vi "Set IP Address.vi"(8 "error in (no error)":errorcluster, 10 "IP Address":string, 11 "ENET in":refnum<class "ENET_BS120x.lvclass">) -> (0 "error out":errorcluster, 3 "ENET out":refnum<class "ENET_BS120x.lvclass">)   [LabVIEW 2021]
uses:
  ENET_BS120x.lvclass
  <vilib>/regexp/Match Regular Expression.xnode
  C:/Users/Public/Documents/Projects/7100-00109 SW BS1201 LV Driver/trunk/source/BS120x.lvclass
  C:/Users/Public/Documents/Projects/7100-00109 SW BS1201 LV Driver/trunk/source/ENET_BS120x/ENET_BS120x.lvclass
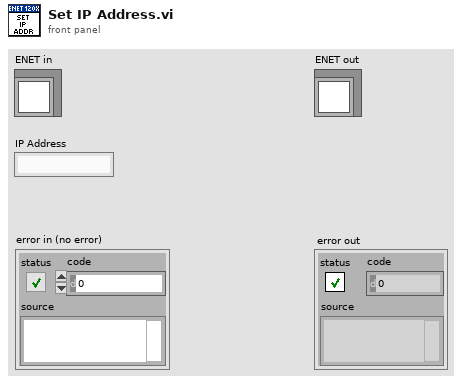
[diagram p1: front panel]
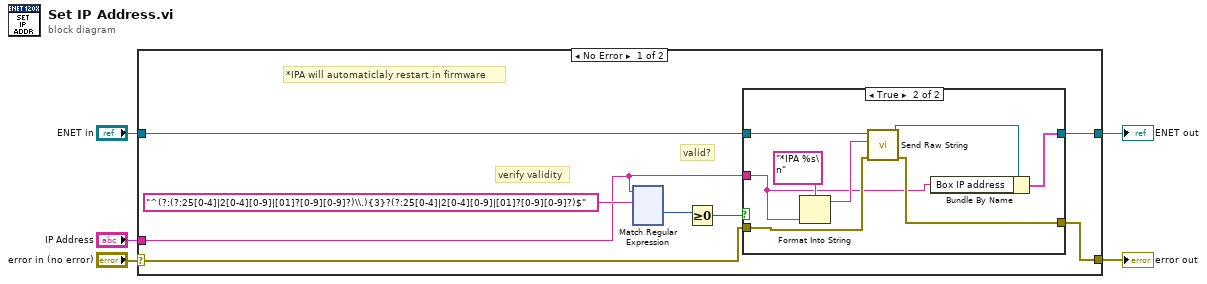
[diagram p0: block diagram]
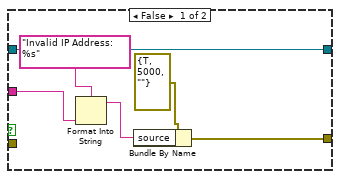
[diagram p2: hidden frame]
diagram:
  n1 = case shown="No Error" "error in (no error)" {
    selector: "error in (no error)" -> [w7 w146]
    tunnel: [w6 w146] -> w5
    tunnel: [w8 w145] -> w4
    tunnel: "ENET in" -> [w13 w145]
    tunnel: "IP Address" -> [w9 _]
    frame No Error {
      # "*IPA will automaticlaly restart in firmware"
      # "valid?"
      # "verify validity"
      n2 = xnode "Match Regular Expression"("input string"=w9, "regular expression"="^(?:(?:25[0-4]|2[0-4][0-9]|[01]?[0-9][0-9]?)\\.){3}?(?:25[0-4]|2[0-4][0-9]|[01]?[0-9][0-9]?)$") -> ("offset past match"=w11:i32)  [unwired: 4 in, 4 out]
      n3 = Greater Or Equal To 0?(x=w11) -> (x >= 0?=w10:bool)
      n4 = case shown="True" w10 {
        tunnel: w13 -> [w19 w27]
        tunnel: w9 -> [w17 w20]
        tunnel: [w19 w21] -> w8
        tunnel: w7 -> [_ w24]
        tunnel: [w14 w23] -> w6
        frame False {
          n5 = Format Into String(format string="Invalid IP Address: %s", w17) -> (resulting string=w15:string)  [unwired: 2 in, 1 out]
          n6 = Bundle By Name(cluster=errorcluster {"status"=TRUE, "code"=5000, "source"=""} ("error out"), "source"=w15) -> (w14:errorcluster)
        }
        frame True {
          n7 = Format Into String(format string="*IPA %s\n", w20) -> (resulting string=w25:string)  [unwired: 2 in, 1 out]
          n8 = call "Send Raw String.vi"("error in (no error)"=w24, "String Data"=w25, "ENET in"=w27) -> ("error out"=w23:errorcluster, "ENET out"=w22:refnum<class "ENET_BS120x.lvclass">)  [unwired: 7 in]
          n9 = Bundle By Name(cluster=w22, "Box IP address"=w20) -> (w21:cluster{})
        }
      }
    }
    frame Error {
    }
  }
  "error out" <- w5
  "ENET out" <- w4
